vi "LiveMovie.vi"() -> ()   [LabVIEW 2024]
doc: "Drag this VI onto your front panel to load several icons that represent working code to display the contents of a movie file."
panel:
  in  "Scrub":i32(slide) scale=1.0..38.0
  in  "Stop":bool
  out "image":picture
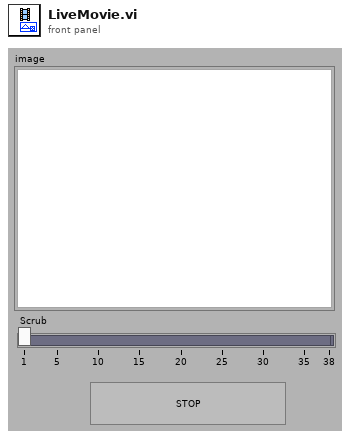
[diagram p1: front panel]
types:
  T1 = typedef "QT_Ref.ctl" = refnum<k1>
  T2 = typedef "QT_Image.ctl" = cluster{"Width":i32, "Height":i32, "Depth":i32, "data":u8[], "Compressed data":u8[], "Color table":u32[], "Duration":i32, "Options":i32, "Timestamp":i32, "ID":i32, "Reserved":i32, "Dialogs":u32}
  T3 = typedef "LVBoundsTypeDef.ctl" = cluster{"Width":u32, "Height":u32}
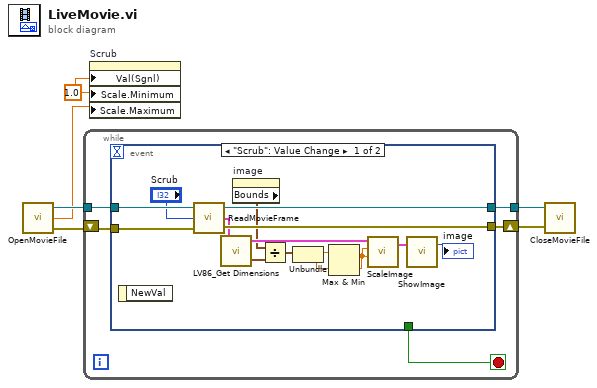
[diagram p0: block diagram]
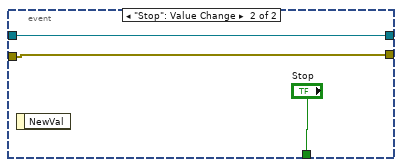
[diagram p2: hidden frame]
diagram:
  w1 = 1.0 ("Scale.Range:Minimum")
  n1 = call <userlib>:"OpenMovieFile.vi"() -> ("error out"=w6:errorcluster, "# frames"=w2:dbl, "QT Ref Out"=w5:T1)  [unwired: 1 in]
  n2 = while {
    tunnel: w5 -> [w10]
    tunnel: [w8] -> w3
    shift-right: [w9] -> w4
    shift-left: w6 -> [w11]
    stop <- w7 stop-if-true
    n3 = event shown="[0] \"Scrub\": Value Change" {
      selector: _ -> [_ _]
      dyn-events: _ -> [_ _]
      timeout: _ -> [_ _]
      tunnel: w11 -> [w26 w27]
      tunnel: w10 -> [w25 w28]
      tunnel: [w24 w27] -> w9
      tunnel: [w23 w28] -> w8
      tunnel: [_ "Stop"] -> w7
      event "Scrub": Value Change {
        n4 = event-data() -> ()  [unwired: 1 in, 1 out]
        n5 = call <userlib>:"ReadMovieFrame.vi"("error in"=w26, "Frame Number"="Scrub", "QT Ref In"=w25) -> ("error out"=w24:errorcluster, "Image Out"=w20:T2, "QT Ref Out"=w23:T1)
        n6 = call <userlib>:"LV86_Get Dimensions.vi"("Image In"=w20) -> ("Dimensions"=w15:cluster{"Width":i32, "Height":i32}, "Image Out"=w19:T2)  [unwired: 1 in]
        n7 = property on="image" class="Pict"() -> ("Bounds"=w16:T3)  [unwired: 2 in, 2 out]
        n8 = Divide(x=w16, y=w15) -> (x/y=w17:cluster{"Width":dbl, "Height":dbl})
        n9 = Unbundle(w17) -> ("Width"=w14:dbl, "Height"=w13:dbl)
        n10 = Max & Min(x=w14, y=w13) -> (min(x,y)=w12:dbl)  [unwired: 1 out]
        n11 = call <userlib>:"ScaleImage.vi"("X scale"=w12, "Y scale"=w12, "Image in"=w19) -> ("Image Out"=w18:T2)  [unwired: 2 in]
        n12 = call <userlib>:"ShowImage.vi"("Image"=w18) -> ("image"=→"image":picture)  [unwired: 2 in, 1 out]
      }
      event "Stop": Value Change {
        n13 = event-data() -> ()  [unwired: 1 in, 1 out]
      }
    }
  }
  n14 = property on="Scrub" class="Slide (strict)"("Val(Sgnl)"=w1, "Scale.Minimum"=w1, "Scale.Maximum"=w2) -> ()  [unwired: 2 in, 2 out]
  n15 = call <userlib>:"CloseMovieFile.vi"("error out"=w4, "QT Ref Out"=w3) -> ()  [unwired: 2 in]
